vi "初始化.vi"(0 "error in (no error)":errorcluster caption="错误输入（无错误）", 3 "数据存储 输入":refnum<class "数据存储.lvclass"> caption="DNL_LabVIEW Object in") -> (7 "error out":errorcluster caption="错误输出", 10 "数据存储 输出":refnum<class "数据存储.lvclass"> caption="DNL_LabVIEW Object out")   [LabVIEW 2013, in "数据存储.lvclass"]
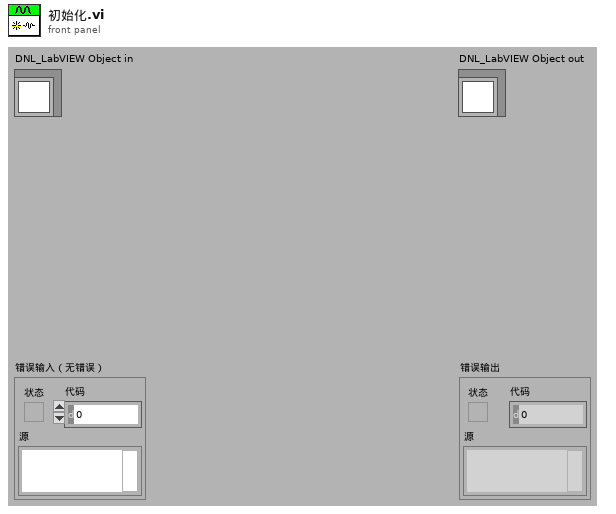
[diagram p1: front panel]
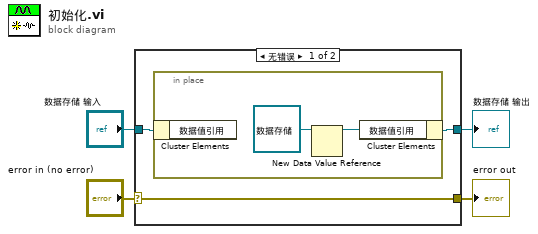
[diagram p0: block diagram]
diagram:
  n1 = case shown="无错误" "error in (no error)" {
    selector: "error in (no error)" -> [w7 w11]
    tunnel: [w7 w11] -> w3
    tunnel: [w5 w10] -> w1
    tunnel: "数据存储 输入" -> [w6 w10]
    frame No Error {
      n2 = in-place {
        n3 = in-place-cluster #1(w6) -> ()  [unwired: 1 out]
        n4 = New Data Value Reference(data value=refnum<class "数据存储.lvclass"> refnum ("数据存储.lvclass")) -> (data value reference=w8:refnum<data-value>)  [unwired: 1 in, 1 out]
        n5 = in-place-cluster #1("数据值引用"=w8) -> (w5:refnum<class "数据存储.lvclass">)
      }
    }
    frame Error {
    }
  }
  "error out" <- w3
  "数据存储 输出" <- w1
